vi "YokoGS200 Set Level.vi"(4 "CtrlRef":refnum<vi>, 6 "RampRate(Unit/s)":dbl=0.005 min=-30.0 max=30.0 step=1e-08, 7 "Ramp":bool, 8 "error in (no error)":errorcluster, 9 "Auto Range":bool, 10 "Output Level":dbl min=-30.0 max=30.0 step=1e-08, 11 "VISA Rsrc":refnum<visa-resource-name>="SR530") -> (0 "error out":errorcluster, 3 "VISA Rsrc Out":refnum<visa-resource-name>="GPIB0::12::INSTR")   [LabVIEW 2012]
uses:
  <userlib>/Yoko GS200/YokoGS200 lvl_states ctl.ctl
panel:
  out "Octet d'état":bool[](array[boolean])
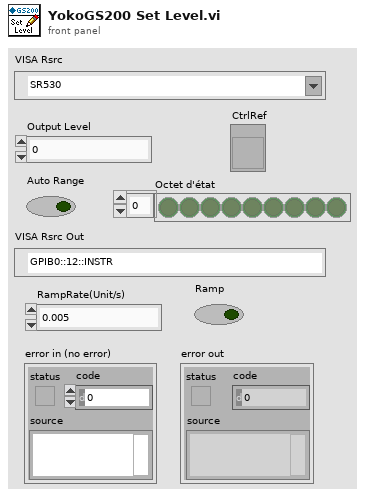
[diagram p1: front panel]
types:
  T1 = typedef "YokoGS200 lvl_states ctl.ctl" = enum16{"RampStep", "Send Command", "Check Errors", "End"}
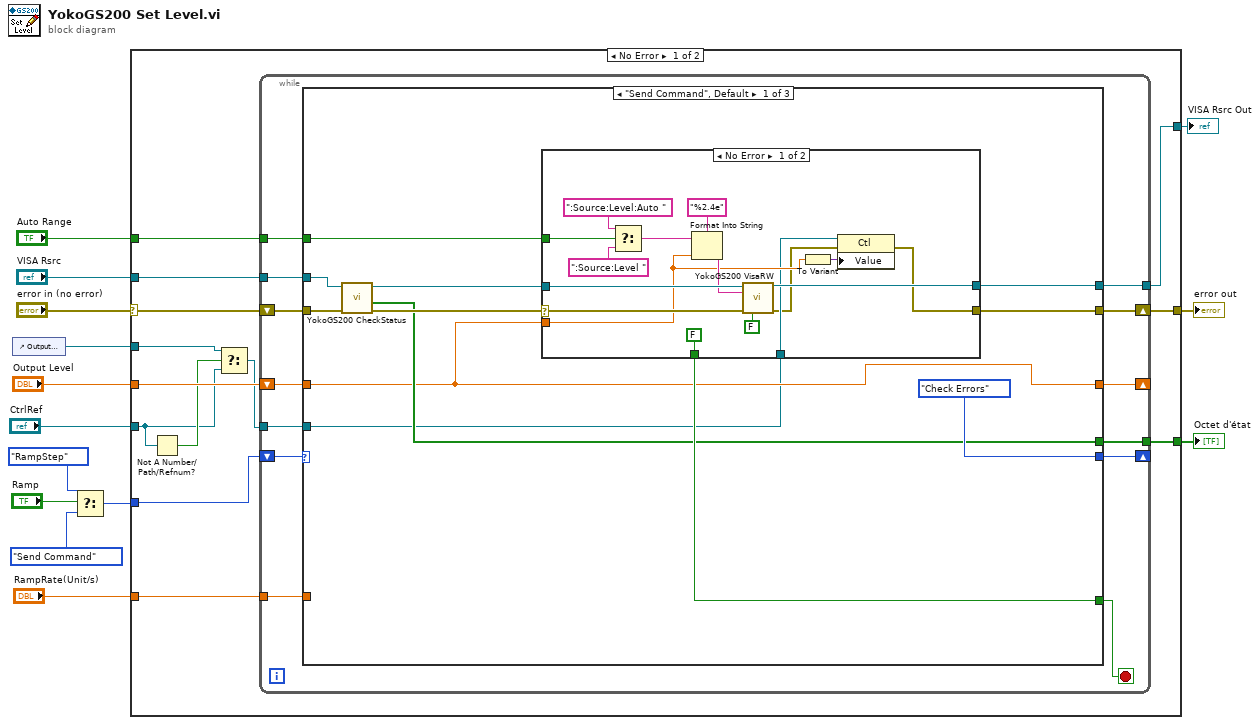
[diagram p0: block diagram]
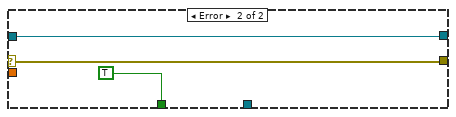
[diagram p2: hidden frame]
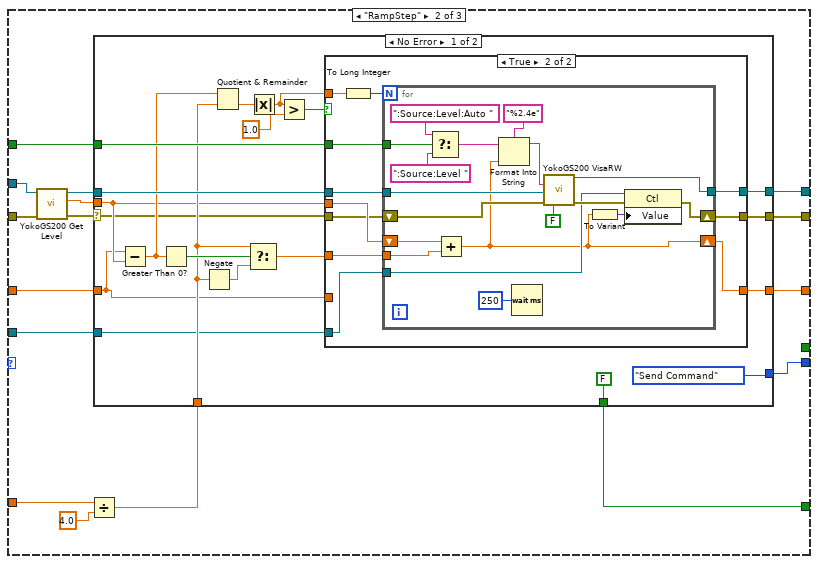
[diagram p3: hidden frame]
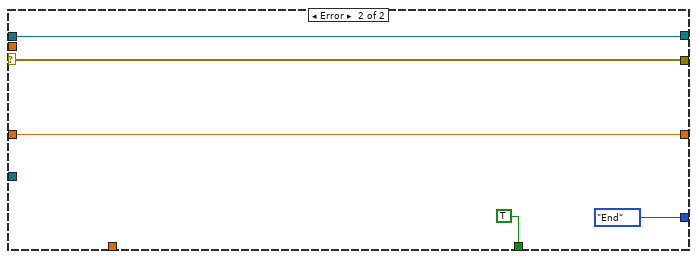
[diagram p5: hidden frame]
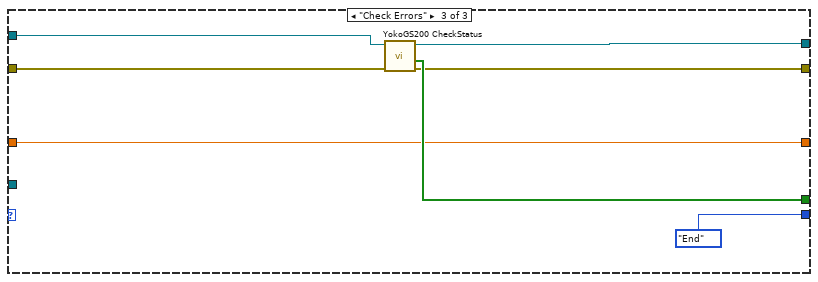
[diagram p6: hidden frame]
diagram:
  n1 = control-ref of="Output Level"() -> (w1:refnum<vi>)
  n2 = Select(t=YokoGS200_lvl_states_ctl."RampStep" ("Level State"), s="Ramp", f=YokoGS200_lvl_states_ctl."Send Command" ("Level State")) -> (s? t:f=w4:T1)
  n3 = case shown="No Error" "error in (no error)" {
    selector: "error in (no error)" -> [w27 w152]
    tunnel: "VISA Rsrc" -> [w26 w153]
    tunnel: [w22 w152] -> w12
    tunnel: [w25 w153] -> w11
    tunnel: "Output Level" -> [w24 _]
    tunnel: "Auto Range" -> [w23 _]
    tunnel: [w21 _] -> w8
    tunnel: w4 -> [w20 _]
    tunnel: "RampRate(Unit/s)" -> [w19 _]
    tunnel: "CtrlRef" -> [w15 _]
    tunnel: w1 -> [w17 _]
    frame No Error {
      n4 = Not A Number/Path/Refnum?(number/path/refnum=w15) -> (NaN/Path/Refnum?=w18:bool)
      n5 = Select(t=w17, s=w18, f=w15) -> (s? t:f=w16:refnum<vi>)
      n6 = while {
        tunnel: w26 -> [w39]
        tunnel: [w38] -> w25
        tunnel: w23 -> [w36]
        shift-right: [w34] -> _
        shift-left: w20 -> [w35]
        shift-right: [w32] -> w22
        shift-left: w27 -> [w40]
        tunnel: [w31] -> w21
        shift-right: [w28] -> _
        shift-left: w24 -> [w37]
        tunnel: w19 -> [w30]
        tunnel: w16 -> [w29]
        stop <- w33 stop-if-true
        n7 = case shown="\"Send Command\", Default" w35 {
          tunnel: w40 -> [w48 w86 w150]
          tunnel: w39 -> [w47 w87 w149]
          tunnel: [w52 w81 w147] -> w38
          tunnel: w37 -> [w42 w78 w145]
          tunnel: [w50 w80 w146] -> w32
          tunnel: w36 -> [w51 w84 _]
          tunnel: [YokoGS200_lvl_states_ctl."Check Errors" ("Level State") w76 YokoGS200_lvl_states_ctl."End" ("Level State")] -> w34
          tunnel: [w44 w75 _] -> w33
          tunnel: [w43 _ w148] -> w31
          tunnel: w30 -> [_ w72 _]
          tunnel: w29 -> [w41 w82 _]
          tunnel: [w42 w79 w145] -> w28
          frame "Send Command", Default {
            n8 = call <userlib>:"YokoGS200 CheckStatus.vi"("error in (no error)"=w48, "VISA Rsrc"=w47) -> ("error out"=w45:errorcluster, "Octet d'état"=w43:bool[], "VISA Rsrc Out"=w46:refnum<visa-resource-name>)  [unwired: 6 in, 1 out]
            n9 = case shown="No Error" w45 {
              selector: w45 -> [w61 w70]
              tunnel: [w68 w69] -> w52
              tunnel: w42 -> [w56 _]
              tunnel: w51 -> [w66 _]
              tunnel: [w53 w70] -> w50
              tunnel: w46 -> [w62 w69]
              tunnel: [FALSE TRUE] -> w44
              tunnel: w41 -> [w55 _]
              frame No Error {
                n10 = Select(t=":Source:Level:Auto " ("initial string"), s=w66, f=":Source:Level " ("initial string")) -> (s? t:f=w63:string)
                n11 = Format Into String(format string="%2.4e", initial string=w63, w56) -> (resulting string=w59:string)  [unwired: 1 in, 1 out]
                n12 = call <userlib>:"YokoGS200 VisaRW.vi"("VISA Rsrc"=w62, "ChaineCom"=w59, "error in (no error)"=w61, "Lecture?(T)"=FALSE) -> ("VISA Rsrc Out"=w68:refnum<visa-resource-name>, "error out"=w54:errorcluster)  [unwired: 7 in, 3 out]
                n13 = To Variant(anything=w56) -> (Variant=w57:variant)
                n14 = property class="Ctl"(reference=w55, error in=w54, "Value"=w57) -> (error out=w53:errorcluster)  [unwired: 1 out]
              }
              frame Error {
              }
            }
          }
          frame "RampStep" {
            n15 = call <userlib>:"YokoGS200 Get Level.vi"("VISA Rsrc"=w87, "error in (no error)"=w86) -> ("VISA Rsrc Out"=w85:refnum<visa-resource-name>, "Output Level"=w83:dbl, "error out"=w77:errorcluster)  [unwired: 6 in]
            n16 = Divide(x=w72, y=4.0 ("x")) -> (x/y=w74:dbl)
            n17 = case shown="No Error" w77 {
              selector: w77 -> [w91 w144]
              tunnel: w85 -> [w105 w143]
              tunnel: w84 -> [w104 _]
              tunnel: w74 -> [w100 _]
              tunnel: w83 -> [w96 _]
              tunnel: w82 -> [w95 _]
              tunnel: [w94 w143] -> w81
              tunnel: [w93 w144] -> w80
              tunnel: [w92 w140] -> w79
              tunnel: w78 -> [w88 w140]
              tunnel: [YokoGS200_lvl_states_ctl."Send Command" ("Level State") YokoGS200_lvl_states_ctl."End" ("Level State")] -> w76
              tunnel: [FALSE TRUE] -> w75
              frame No Error {
                n18 = Subtract(x=w88, y=w96) -> (x-y=w101:dbl)
                n19 = Greater Than 0?(x=w101) -> (x > 0?=w107:bool)
                n20 = Negate(x=w100) -> (-x=w106:dbl)
                n21 = Quotient & Remainder(x=w101, y=w100) -> (floor(x/y)=w103:dbl)  [unwired: 1 out]
                n22 = Select(t=w100, s=w107, f=w106) -> (s? t:f=w97:dbl)
                n23 = Absolute Value(x=w103) -> (abs(x)=w98:dbl)
                n24 = Greater?(x=w98, y=1.0) -> (0:w99:bool)
                n25 = case shown="True" w99 {
                  tunnel: [w110 w121] -> w94
                  tunnel: w104 -> [_ w120]
                  tunnel: [w109 w119] -> w93
                  tunnel: w105 -> [w110 w118]
                  tunnel: w91 -> [w109 w113]
                  tunnel: w98 -> [_ w117]
                  tunnel: w97 -> [_ w115]
                  tunnel: w96 -> [_ w114]
                  tunnel: w95 -> [_ w112]
                  tunnel: [w108 w111] -> w92
                  tunnel: w88 -> [w108 _]
                  frame False {
                  }
                  frame True {
                    n26 = To Long Integer(number=w117) -> (32bit integer=w116:i32)
                    n27 = for {
                      N: w116 -> [_]
                      tunnel: [w128] -> w121
                      tunnel: w120 -> [w138]
                      tunnel: w118 -> [w134]
                      tunnel: w115 -> [w131]
                      shift-right: [w123] -> w111
                      shift-left: w114 -> [w130]
                      shift-right: [w126] -> w119
                      shift-left: w113 -> [w129]
                      tunnel: w112 -> [w125]
                      n28 = Select(t=":Source:Level:Auto " ("initial string"), s=w138, f=":Source:Level " ("initial string")) -> (s? t:f=w135:string)
                      n29 = Add(x=w130, y=w131) -> (x+y=w123:dbl)
                      n30 = Format Into String(format string="%2.4e", initial string=w135, w123) -> (resulting string=w133:string)  [unwired: 1 in, 1 out]
                      n31 = Wait (ms)(milliseconds to wait=u32 250) -> ()  [unwired: 1 out]
                      n32 = call <userlib>:"YokoGS200 VisaRW.vi"("VISA Rsrc"=w134, "ChaineCom"=w133, "error in (no error)"=w129, "Lecture?(T)"=FALSE) -> ("VISA Rsrc Out"=w128:refnum<visa-resource-name>, "error out"=w127:errorcluster)  [unwired: 7 in, 3 out]
                      n33 = To Variant(anything=w123) -> (Variant=w124:variant)
                      n34 = property class="Ctl"(reference=w125, error in=w127, "Value"=w124) -> (error out=w126:errorcluster)  [unwired: 1 out]
                    }
                  }
                }
              }
              frame Error {
              }
            }
          }
          frame "Check Errors" {
            n35 = call <userlib>:"YokoGS200 CheckStatus.vi"("error in (no error)"=w150, "VISA Rsrc"=w149) -> ("error out"=w146:errorcluster, "Octet d'état"=w148:bool[], "VISA Rsrc Out"=w147:refnum<visa-resource-name>)  [unwired: 6 in, 1 out]
          }
        }
      }
    }
    frame Error {
    }
  }
  "error out" <- w12
  "VISA Rsrc Out" <- w11
  "Octet d'état" <- w8
